vi "I2C Device Write.vi"(0 "handle":u32, 5 "deviceAddress":u32, 7 "Data to write":u8[](array[numeric]) format="%.0x", 9 "options":T1, 11 "error in (no error)":errorcluster) -> (4 "handle out":u32, 6 "sizeTransfered":u32, 15 "error out":errorcluster)   [LabVIEW 2017, in "libMPSSE.lvlib"]
doc: "FTDI_API FT_STATUS I2C_DeviceWrite(FT_HANDLE handle, uint32 deviceAddress, \nuint32 sizeToTransfer, uint8 *buffer, uint32 *sizeTransfered, uint32 options);\n\n\nOptions\nThis parameter specifies data transfer options. The bit positions defined for each of these options are:\n\nBIT0: if set then a start condition is generated in the I2C bus before the transfer begins. A bit mask is defined for this options in file ftdi_i2c.h as I2C_TRANSFER_OPTIONS_START_BIT\n\nBIT1: if set then a stop condition is generated in the I2C bus after the transfer ends. A bit mask is defined for this options in file ftdi_i2c.h as I2C_TRANSFER_OPTIONS_STOP_BIT\n\nBIT2: if set then the function will return when a device nAcks after a byte has been transferred. If not set then the function will continue transferring the stream of bytes even if the device nAcks. A bit mask is defined for this options in file ftdi_i2c.h as I2C_TRANSFER_OPTIONS_BREAK_ON_NACK\n\nBIT3: reserved (only used in I2C_DeviceRead)\n\nBIT4: setting this bit will invoke a multi byte I2C\nApplication Note: AN_177 User Guide For libMPSSE – I2C Version 1.4 Document Reference No.: FT_000466 Clearance No.: FTDI# 210 11 Copyright © 2011 Future Technology Devices International Limited\ntransfer without having delays between the START, ADDRESS, DATA and STOP phases. Size of the transfer in parameters sizeToTransfer and sizeTransfered are in bytes. The bit mask defined for this bit is I2C_TRANSFER_OPTIONS_FAST_TRANSFER_BYTES*\n\nBIT5: setting this bit would invoke a multi bit transfer without having delays between the START, ADDRESS, DATA and STOP phases. Size of the transfer in parameters sizeToTransfer and sizeTransfered are in bytes. The bit mask defined for this bit is I2C_TRANSFER_OPTIONS_FAST_TRANSFER_BITS*\n\nBIT6: the deviceAddress parameter is ignored if this bit is set. This feature may be useful in generating a special I2C bus conditions that do not require any address to be passed.Setting this bit is effective only when either I2C_TRANSFER_OPTIONS_FAST_TRANSFER_BYTES or I2C_TRANSFER_OPTIONS_FAST_TRANSFER_BITS is set. The bit mask defined for this bit is I2C_TRANSFER_OPTIONS_NO_ADDRESS*\n\nBIT7 – BIT31: reserved"
uses:
  libMPSSE.lvlib
  libMPSSE-SPI-LabVIEW-master/libMPSSE.dll
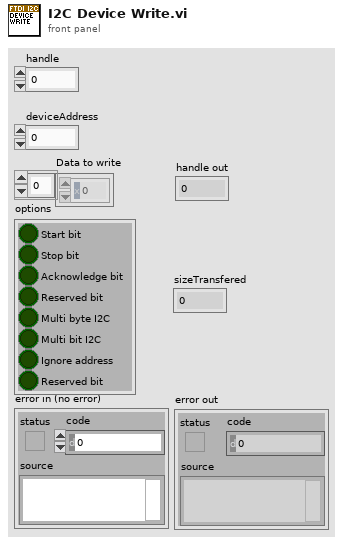
[diagram p1: front panel]
types:
  T1 = cluster{"Start bit":bool, "Stop bit":bool, "Acknowledge bit":bool, "Reserved bit":bool, "Multi byte I2C":bool, "Multi bit I2C":bool, "Ignore address":bool, "Reserved bit":bool}
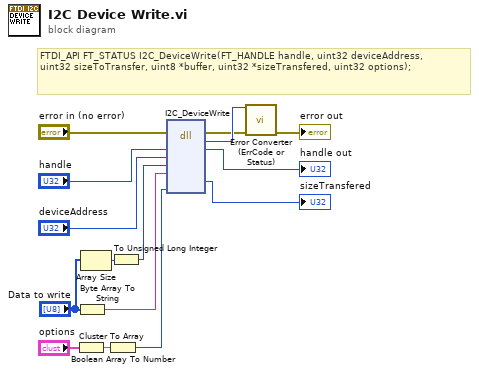
[diagram p0: block diagram]
diagram:
  # "FTDI_API FT_STATUS I2C_DeviceWrite(FT_HANDLE handle, uint32 deviceAddress, \nuint32 sizeToTransfer, uint8 *buffer, uint32 *sizeTransfered, uint32 options);"
  n1 = Cluster To Array(cluster="options") -> (array=w6:bool[])
  n2 = Byte Array To String(unsigned byte array="Data to write") -> (string=w4:string)
  n3 = Array Size(array="Data to write") -> (size(s)=w2:i32)
  n4 = Boolean Array To Number(Boolean array=w6) -> (number=w5:u32)
  n5 = To Unsigned Long Integer(number=w2) -> (unsigned 32bit integer=w1:u32)
  n6 = dll-call lib="\\\\Mac\\Home/Desktop/libMPSSE-SPI-LabVIEW-master/libMPSSE.dll" fn="I2C_DeviceWrite"(error in="error in (no error)", "handle"="handle", "deviceAddress"="deviceAddress", "sizeToTransfer"=w1, "buffer"=w4, "options"=w5) -> (error out=w9:errorcluster, "return type"=w15:u32, "handle"=→"handle out":u32, "sizeTransfered"=→"sizeTransfered":u32)  [unwired: 7 in, 1 out]
  n7 = call "Error Converter (ErrCode or Status).vi"("error code"=w15, "error in (no error)"=w9) -> ("error out"=→"error out":errorcluster)  [unwired: 13 in]
